vi "Copy PPLs to Includes.vi"(5 "Files Generated by Build":path[](array[path]), 6 "Top Level/Always Included VIs":path[](array[path]), 7 "Destination Path":path, 8 "error in":errorcluster, 9 "Target Name":string, 10 "Build Specification Name":string, 11 "Project Path":path) -> (0 "error out":errorcluster)   [LabVIEW 2020]
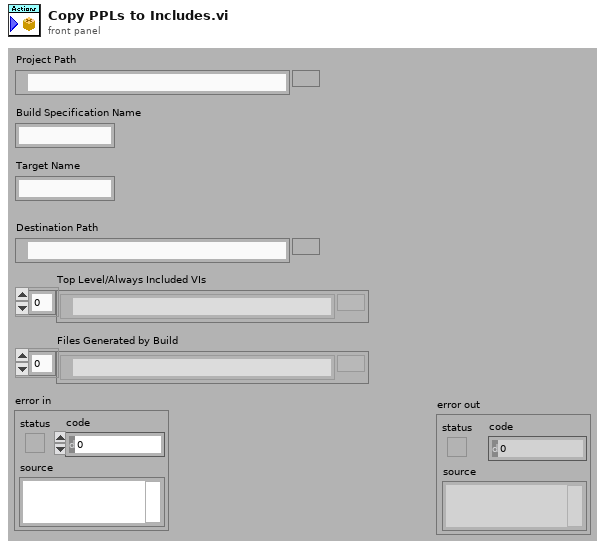
[diagram p1: front panel]
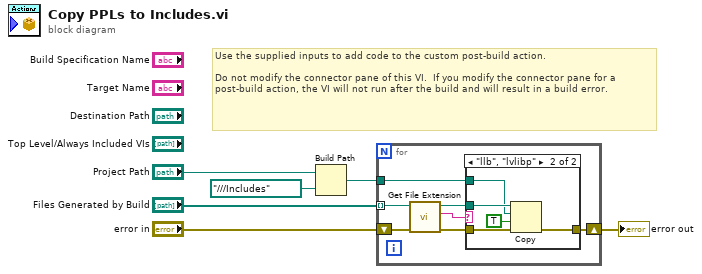
[diagram p0: block diagram]
diagram:
  # "Use the supplied inputs to add code to the custom post-build action.\n\nDo not modify the connector pane of this VI.  If you modify the connector pane for a post-build action, the VI will not run after the build and will result in a build error."
  n1 = Build Path(base path="Project Path", name or relative path=path "../../../Includes") -> (appended path=w1:path)
  n2 = for {
    shift-right: [w10] -> w5
    shift-left: "error in" -> [w13]
    tunnel: "Files Generated by Build" -> [w12] mode=indexing
    tunnel: w1 -> [w8]
    n3 = call <vilib>:"Get File Extension.vi"("error in (no error)"=w13, "file"=w12) -> ("error out"=w11:errorcluster, "lowercase file extension"=w7:string, "dup file"=w9:path)  [unwired: 5 in, 2 out]
    n4 = case shown="\"llb\", \"lvlibp\"" w7 {
      tunnel: w11 -> [w14 w19]
      tunnel: [w14 w18] -> w10
      tunnel: w9 -> [_ w16]
      tunnel: w8 -> [_ w15]
      frame Default {
      }
      frame "llb", "lvlibp" {
        n5 = Copy(8:w19, 9:TRUE ("overwrite (F)"), 10:w15, 11:w16) -> (0:w18:errorcluster)  [unwired: 1 in, 2 out]
      }
    }
  }
  "error out" <- w5
